vi "Remove Double Quotes from String (Util).vi"(11 "String In":string) -> (3 "Quotes Removed":string)   [LabVIEW 2019]
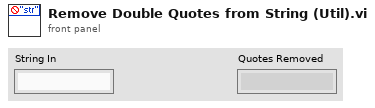
[diagram p1: front panel]
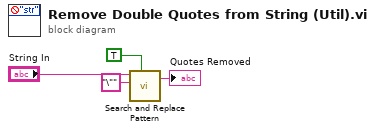
[diagram p0: block diagram]
diagram:
  n1 = call <vilib>:"Search and Replace Pattern.vi"("string"="String In", "regular expression (\"\")"="\"" ("regular expression (\"\")"), "replace all? (F)"=TRUE) -> ("result string"=→"Quotes Removed":string)  [unwired: 2 in, 1 out]
